vi "Destroy User Event - Stop.vi"(8 "Error In":errorcluster) -> (0 "Error Out":errorcluster)   [LabVIEW 2017]
doc: "Destroy the user event, even if there is an incoming error."
uses:
  Global Variables/gl_User Events.vi
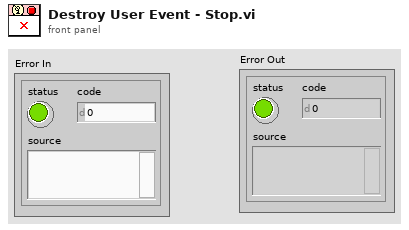
[diagram p1: front panel]
types:
  T1 = cluster{"User Event - Stop":refnum<user-event>, "User Event - Next State":refnum<user-event>}
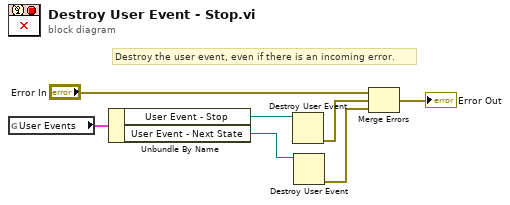
[diagram p0: block diagram]
diagram:
  # "Destroy the user event, even if there is an incoming error."
  n1 = global read "gl_User Events.vi" "User Events"() -> (w4:T1)
  n2 = Unbundle By Name(w4) -> ("User Event - Stop"=w3:refnum<user-event>, "User Event - Next State"=w1:refnum<user-event>)
  n3 = Destroy User Event(user event=w3) -> (error out=w7:errorcluster)  [unwired: 1 in]
  n4 = Destroy User Event(user event=w1) -> (error out=w2:errorcluster)  [unwired: 1 in]
  n5 = Merge Errors("Error In", w7, w2) -> (→"Error Out":errorcluster)
